vi "Convert Excel To 2D Data.vi"(8 "error in (no error)":errorcluster, 9 "SheetName(\"\")":string="测试", 10 "Path":path, 11 "ExcelReader in":refnum<class "ExcelReader.lvclass">) -> (0 "error out":errorcluster, 2 "data":string[][](array[string]), 3 "ExcelReader out":refnum<class "ExcelReader.lvclass">)   [LabVIEW 2015, in "Admin_Actor.lvlib" / "ExcelReader.lvclass"]
uses:
  ExcelReader.lvclass
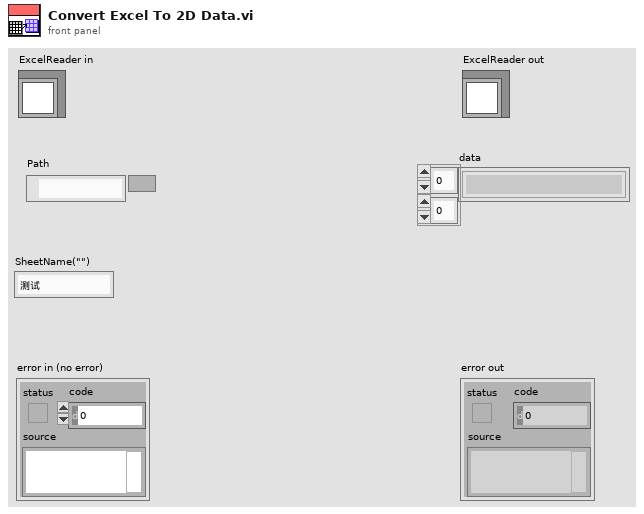
[diagram p1: front panel]
types:
  T1 = cluster{"Excel._Application":refnum<k7>, "Workbooks":refnum<k7>}
  T2 = cluster{"Excel._Application":refnum<k7>, "Workbooks":refnum<k7>, "Open":refnum<k7>}
  T3 = cluster{"Excel._Application":refnum<k7>, "Workbooks":refnum<k7>, "Open":refnum<k7>, "Worksheets":refnum<k7>, "Excel._Worksheet":refnum<k7>}
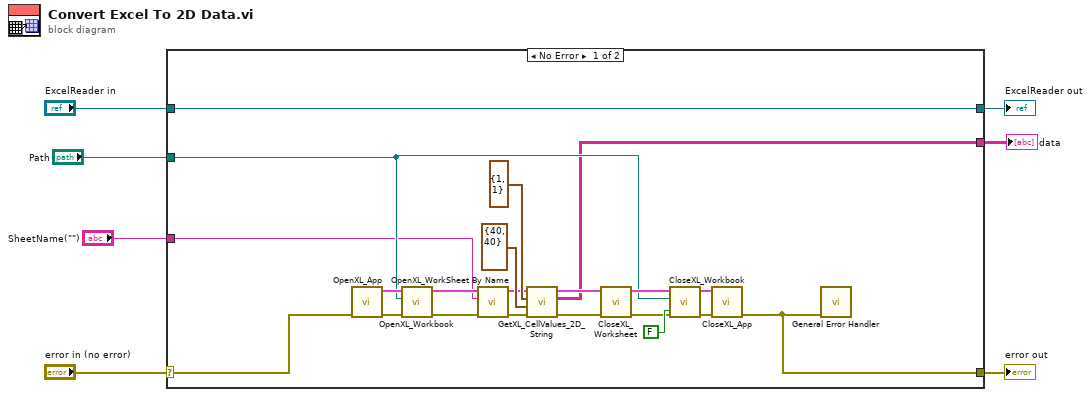
[diagram p0: block diagram]
diagram:
  n1 = case shown="No Error" "error in (no error)" {
    selector: "error in (no error)" -> [w11 w30]
    tunnel: [w10 w30] -> w6
    tunnel: [w28 w29] -> w4
    tunnel: "ExcelReader in" -> [w28 w29]
    tunnel: "Path" -> [w12 _]
    tunnel: "SheetName(\"\")" -> [w9 _]
    tunnel: [w8 _] -> w1
    frame No Error {
      n2 = call "OpenXL_App.vi"("error in (no error)"=w11) -> ("error out"=w14:errorcluster, "Refnum Cluster"=w13:T1)  [unwired: 9 in]
      n3 = call "OpenXL_Workbook.vi"("error in"=w14, "path"=w12, "Refnum Cluster In"=w13) -> ("error out"=w21:errorcluster, "Refnum Cluster Out"=w20:T2)  [unwired: 7 in]
      n4 = call "OpenXL_WorkSheet By Name.vi"("error in (no error)"=w21, "SheetName(\"\")"=w9, "Refnum Cluster In"=w20) -> ("error out"=w23:errorcluster, "Refnum Cluster Out"=w22:T3)  [unwired: 7 in]
      n5 = call "GetXL_CellValues_2D_String.vi"("error in"=w23, "End"=cluster{"Column":i32, "Row":i32} {"Column"=40, "Row"=40}, "Start"=cluster{"Column":i32, "Row":i32} {"Column"=1, "Row"=1}, "Refnum Cluster In"=w22) -> ("error out"=w27:errorcluster, "data"=w8:string[][], "Refnum Cluster Out"=w26:T3)  [unwired: 5 in]
      n6 = call "CloseXL_Worksheet.vi"("error in (no error)"=w27, "Refnum Cluster In"=w26) -> ("error out"=w15:errorcluster, "Refnum Cluster Out"=w16:T2)  [unwired: 8 in]
      n7 = call "CloseXL_Workbook.vi"("Save? (F)"=FALSE, "error in (no error)"=w15, "path"=w12, "Refnum Cluster In"=w16) -> ("error out"=w17:errorcluster, "Refnum Cluster Out"=w18:T1)  [unwired: 6 in]
      n8 = call "CloseXL_App.vi"("error in (no error)"=w17, "Refnum Cluster In"=w18) -> ("error out"=w10:errorcluster)  [unwired: 9 in]
      n9 = call <vilib>:"General Error Handler.vi"("error in (no error)"=w10) -> ()  [unwired: 10 in, 5 out]
    }
    frame Error {
    }
  }
  "error out" <- w6
  "ExcelReader out" <- w4
  "data" <- w1
